vi "Single Slow IV v1.4.vi"() -> ()   [LabVIEW 2020]
uses:
  <vilib>/Utility/file.llb/Write Delimited Spreadsheet (DBL).vi
panel:
  out "Current variable":dbl
  in  "stop":bool
  in  "Tab Control 2":enum32{"cRIO plot", "Lockin X", "Lockin Y"}(tab)
  out "cRIO data plot":cluster{"Y":dbl[], "Y":dbl[]}[](graph)=[{"Y"=[0.1, 0.101, 0.10200000000000001, 0.10300000000000001, 0.10400000000000001, 0.10500000000000001, 0.10600000000000001, 0.10700000000000001, 0.10800000000000001, 0.10900000000000001, 0.11, 0.111, 0.112, 0.113, 0.114, 0.115, 0.116, 0.117, 0.11800000000000001, 0.11900000000000001, 0.12000000000000001, 0.12100000000000001, 0.122, 0.123, 0.124, 0.125, 0.126, 0.127, 0.128, 0.129, 0.13, 0.131, 0.132, 0.133, 0.134, 0.135, 0.136, 0.137, 0.138, 0.139, 0.14, 0.14100000000000001, 0.14200000000000002, 0.14300000000000002, 0.14400000000000002, 0.14500000000000002, 0.14600000000000002, 0.14700000000000002, 0.14800000000000002, 0.14900000000000002, 0.15000000000000002, 0.15100000000000002, 0.15200000000000002, 0.153, 0.154, 0.155, 0.156, 0.157, 0.158, 0.159, 0.16, 0.161, 0.162, 0.163, 0.164, 0.165, 0.166, 0.167, 0.168, 0.169, 0.17, 0.171, 0.17200000000000001, 0.173, 0.174, 0.175, 0.176, 0.177, 0.178, 0.179, 0.18, 0.181, 0.182, 0.183, 0.184, 0.185, 0.186, 0.187, 0.188, 0.189, 0.19, 0.191, 0.192, 0.193, 0.194, 0.195, 0.196, 0.197, 0.198, 0.199, 0.2], "Y"=[1.91443115234375e-05, 1.8234204101562503e-05, 1.8079296875e-05, 1.72965576171875e-05, 1.73908447265625e-05, 1.6982641601562502e-05, 1.7475024414062502e-05, 1.7350537109375e-05, 1.80681884765625e-05, 1.8036865234375e-05, 1.8520703124999998e-05, 1.9111669921875e-05, 1.948046875e-05, 1.9645117187500002e-05, 1.95529296875e-05, 1.9983398437500002e-05, 1.99129638671875e-05, 1.99599365234375e-05, 1.8666650390625e-05, 1.8764892578125e-05, 1.78889892578125e-05, 1.7660498046875002e-05, 1.7441210937500002e-05, 1.69652587890625e-05, 1.67341064453125e-05, 1.5950341796875e-05, 1.6491918945312503e-05, 1.61111572265625e-05, 1.6419482421875e-05, 1.6167163085937502e-05, 1.6684667968750002e-05, 1.66596923828125e-05, 1.76610595703125e-05, 1.7373608398437503e-05, 1.7419580078125e-05, 1.7511450195312502e-05, 1.76984619140625e-05, 1.7275e-05, 1.8423168945312502e-05, 1.78859619140625e-05, 1.74806396484375e-05, 1.7222802734375003e-05, 1.6946435546875e-05, 1.5935034179687498e-05, 1.5810864257812502e-05, 1.527841796875e-05, 1.509169921875e-05, 1.4530908203125001e-05, 1.4473876953125001e-05, 1.4885107421875e-05, 1.4928662109374999e-05, 1.5158349609375e-05, 1.5753149414062502e-05, 1.6247314453125003e-05, 1.59515625e-05, 1.62923583984375e-05, 1.64744873046875e-05, 1.65873779296875e-05, 1.7040673828125e-05, 1.65896484375e-05, 1.76021484375e-05, 1.6583422851562498e-05, 1.6492236328125e-05, 1.5975390625e-05, 1.57067138671875e-05, 1.4773681640625001e-05, 1.5178466796875001e-05, 1.4151171875e-05, 1.4718139648437501e-05, 1.453740234375e-05, 1.45205322265625e-05, 1.39417724609375e-05, 1.42656982421875e-05, 1.4501342773437501e-05, 1.4439892578125e-05, 1.47739501953125e-05, 1.47328369140625e-05, 1.46720703125e-05, 1.51514404296875e-05, 1.5362841796875e-05, 1.5647558593750002e-05, 1.612255859375e-05, 1.57461181640625e-05, 1.56584716796875e-05, 1.5264282226562502e-05, 1.4975024414062499e-05, 1.4608837890625003e-05, 1.4593286132812501e-05, 1.44783935546875e-05, 1.40139404296875e-05, 1.36931640625e-05, 1.3610986328125e-05, 1.3888769531250001e-05, 1.35940673828125e-05, 1.35070068359375e-05, 1.3863745117187502e-05, 1.45044677734375e-05, 1.418330078125e-05, 1.45068115234375e-05, 1.4514819335937501e-05, 1.4418505859375001e-05]}, {"Y"=[0.1, 0.101, 0.10200000000000001, 0.10300000000000001, 0.10400000000000001, 0.10500000000000001, 0.10600000000000001, 0.10700000000000001, 0.10800000000000001, 0.10900000000000001, 0.11, 0.111, 0.112, 0.113, 0.114, 0.115, 0.116, 0.117, 0.11800000000000001, 0.11900000000000001, 0.12000000000000001, 0.12100000000000001, 0.122, 0.123, 0.124, 0.125, 0.126, 0.127, 0.128, 0.129, 0.13, 0.131, 0.132, 0.133, 0.134, 0.135, 0.136, 0.137, 0.138, 0.139, 0.14, 0.14100000000000001, 0.14200000000000002, 0.14300000000000002, 0.14400000000000002, 0.14500000000000002, 0.14600000000000002, 0.14700000000000002, 0.14800000000000002, 0.14900000000000002, 0.15000000000000002, 0.15100000000000002, 0.15200000000000002, 0.153, 0.154, 0.155, 0.156, 0.157, 0.158, 0.159, 0.16, 0.161, 0.162, 0.163, 0.164, 0.165, 0.166, 0.167, 0.168, 0.169, 0.17, 0.171, 0.17200000000000001, 0.173, 0.174, 0.175, 0.176, 0.177, 0.178, 0.179, 0.18, 0.181, 0.182, 0.183, 0.184, 0.185, 0.186, 0.187, 0.188, 0.189, 0.19, 0.191, 0.192, 0.193, 0.194, 0.195, 0.196, 0.197, 0.198, 0.199, 0.2], "Y"=[2.07511962890625, 2.0750732421875, 2.074141357421875, 2.075462646484375, 2.075708740234375, 2.074308349609375, 2.074795654296875, 2.07555810546875, 2.0755185546875, 2.07468310546875, 2.074645751953125, 2.074962646484375, 2.0738427734375, 2.074322509765625, 2.07427294921875, 2.074574951171875, 2.075367431640625, 2.07494384765625, 2.074665771484375, 2.074663330078125, 2.07564013671875, 2.074562255859375, 2.074658935546875, 2.074733154296875, 2.07546826171875, 2.074733154296875, 2.074750244140625, 2.07523779296875, 2.07525244140625, 2.074369384765625, 2.075072265625, 2.0747587890625, 2.075584228515625, 2.075943603515625, 2.074529541015625, 2.07461474609375, 2.075067138671875, 2.075061279296875, 2.07536279296875, 2.07553466796875, 2.074748779296875, 2.075227294921875, 2.074936279296875, 2.075556396484375, 2.0753974609375, 2.0758994140625, 2.0761806640625, 2.075328369140625, 2.07436767578125, 2.076673828125, 2.076259765625, 2.075400146484375, 2.075468505859375, 2.075495849609375, 2.076040283203125, 2.0754658203125, 2.075578125, 2.0752451171875, 2.07488134765625, 2.07554736328125, 2.0753955078125, 2.0752822265625, 2.075176513671875, 2.076365478515625, 2.076373046875, 2.076056884765625, 2.07583837890625, 2.075223388671875, 2.0750703125, 2.07514599609375, 2.075769775390625, 2.0751220703125, 2.07619775390625, 2.075202392578125, 2.075671630859375, 2.07513916015625, 2.076079345703125, 2.076094970703125, 2.075864501953125, 2.07488134765625, 2.07613525390625, 2.076350341796875, 2.07625, 2.07523876953125, 2.075680419921875, 2.0746162109375, 2.076003173828125, 2.0753193359375, 2.075281494140625, 2.0755927734375, 2.075462158203125, 2.07468505859375, 2.07553564453125, 2.075280517578125, 2.0758173828125, 2.075341796875, 2.07434033203125, 2.074906005859375, 2.074229248046875, 2.0753671875, 2.0744853515625]}, {"Y"=[0.1, 0.101, 0.10200000000000001, 0.10300000000000001, 0.10400000000000001, 0.10500000000000001, 0.10600000000000001, 0.10700000000000001, 0.10800000000000001, 0.10900000000000001, 0.11, 0.111, 0.112, 0.113, 0.114, 0.115, 0.116, 0.117, 0.11800000000000001, 0.11900000000000001, 0.12000000000000001, 0.12100000000000001, 0.122, 0.123, 0.124, 0.125, 0.126, 0.127, 0.128, 0.129, 0.13, 0.131, 0.132, 0.133, 0.134, 0.135, 0.136, 0.137, 0.138, 0.139, 0.14, 0.14100000000000001, 0.14200000000000002, 0.14300000000000002, 0.14400000000000002, 0.14500000000000002, 0.14600000000000002, 0.14700000000000002, 0.14800000000000002, 0.14900000000000002, 0.15000000000000002, 0.15100000000000002, 0.15200000000000002, 0.153, 0.154, 0.155, 0.156, 0.157, 0.158, 0.159, 0.16, 0.161, 0.162, 0.163, 0.164, 0.165, 0.166, 0.167, 0.168, 0.169, 0.17, 0.171, 0.17200000000000001, 0.173, 0.174, 0.175, 0.176, 0.177, 0.178, 0.179, 0.18, 0.181, 0.182, 0.183, 0.184, 0.185, 0.186, 0.187, 0.188, 0.189, 0.19, 0.191, 0.192, 0.193, 0.194, 0.195, 0.196, 0.197, 0.198, 0.199, 0.2], "Y"=[0.000849365234375, 0.0008095703125, 0.000814453125, 0.00078076171875, 0.000771240234375, 0.000831787109375, 0.000755859375, 0.00079150390625, 0.0008310546875, 0.00079150390625, 0.00074560546875, 0.00078369140625, 0.000753662109375, 0.00079296875, 0.0007275390625, 0.000805419921875, 0.00074658203125, 0.00084375, 0.000741943359375, 0.00080859375, 0.00072705078125, 0.0007802734375, 0.0007021484375, 0.0008046875, 0.000873779296875, 0.000772216796875, 0.0007861328125, 0.000777587890625, 0.00078466796875, 0.00077001953125, 0.000764404296875, 0.0007626953125, 0.000732421875, 0.00077783203125, 0.00079150390625, 0.0007861328125, 0.000770751953125, 0.0008134765625, 0.00080419921875, 0.00079345703125, 0.000803466796875, 0.0007470703125, 0.000757080078125, 0.000783935546875, 0.000799072265625, 0.000781982421875, 0.00076904296875, 0.000742919921875, 0.00082666015625, 0.00078369140625, 0.000858154296875, 0.00076318359375, 0.0006982421875, 0.00071728515625, 0.00077099609375, 0.00078076171875, 0.000766845703125, 0.00076806640625, 0.000752197265625, 0.000720703125, 0.00075830078125, 0.00077099609375, 0.0008076171875, 0.000795166015625, 0.00074365234375, 0.000795166015625, 0.00078125, 0.000791748046875, 0.000809814453125, 0.00074755859375, 0.000774658203125, 0.000756103515625, 0.00083251953125, 0.000758056640625, 0.00082470703125, 0.00077197265625, 0.000834228515625, 0.000770751953125, 0.00077734375, 0.000760009765625, 0.000823974609375, 0.00071533203125, 0.000766357421875, 0.0007548828125, 0.000796630859375, 0.000743408203125, 0.000770751953125, 0.000744384765625, 0.0007314453125, 0.000734130859375, 0.000804443359375, 0.0007275390625, 0.000815673828125, 0.000766357421875, 0.000784912109375, 0.000762451171875, 0.00075, 0.000779296875, 0.000757080078125, 0.000751953125, 0.000764892578125]}, {"Y"=[0.1, 0.101, 0.10200000000000001, 0.10300000000000001, 0.10400000000000001, 0.10500000000000001, 0.10600000000000001, 0.10700000000000001, 0.10800000000000001, 0.10900000000000001, 0.11, 0.111, 0.112, 0.113, 0.114, 0.115, 0.116, 0.117, 0.11800000000000001, 0.11900000000000001, 0.12000000000000001, 0.12100000000000001, 0.122, 0.123, 0.124, 0.125, 0.126, 0.127, 0.128, 0.129, 0.13, 0.131, 0.132, 0.133, 0.134, 0.135, 0.136, 0.137, 0.138, 0.139, 0.14, 0.14100000000000001, 0.14200000000000002, 0.14300000000000002, 0.14400000000000002, 0.14500000000000002, 0.14600000000000002, 0.14700000000000002, 0.14800000000000002, 0.14900000000000002, 0.15000000000000002, 0.15100000000000002, 0.15200000000000002, 0.153, 0.154, 0.155, 0.156, 0.157, 0.158, 0.159, 0.16, 0.161, 0.162, 0.163, 0.164, 0.165, 0.166, 0.167, 0.168, 0.169, 0.17, 0.171, 0.17200000000000001, 0.173, 0.174, 0.175, 0.176, 0.177, 0.178, 0.179, 0.18, 0.181, 0.182, 0.183, 0.184, 0.185, 0.186, 0.187, 0.188, 0.189, 0.19, 0.191, 0.192, 0.193, 0.194, 0.195, 0.196, 0.197, 0.198, 0.199, 0.2], "Y"=[0.00172021484375, 0.001699462890625, 0.001721435546875, 0.001740966796875, 0.001722412109375, 0.001780517578125, 0.001792724609375, 0.00180224609375, 0.001711181640625, 0.00181494140625, 0.001773193359375, 0.001771240234375, 0.00173388671875, 0.001708740234375, 0.00180908203125, 0.001841064453125, 0.001756103515625, 0.00170068359375, 0.00175, 0.001714111328125, 0.001801025390625, 0.001765625, 0.0017099609375, 0.001703857421875, 0.001786865234375, 0.0018046875, 0.001700927734375, 0.001765380859375, 0.001693603515625, 0.00175244140625, 0.0017626953125, 0.0017978515625, 0.001715576171875, 0.001716064453125, 0.00177099609375, 0.00180712890625, 0.001722900390625, 0.001816650390625, 0.001749755859375, 0.00174755859375, 0.001776123046875, 0.00170849609375, 0.00172509765625, 0.001736083984375, 0.00171533203125, 0.001705322265625, 0.001744873046875, 0.001779296875, 0.001696044921875, 0.00173974609375, 0.001815185546875, 0.001720947265625, 0.00178076171875, 0.001763916015625, 0.0017958984375, 0.0017158203125, 0.00179248046875, 0.001754638671875, 0.00173193359375, 0.001706298828125, 0.00173388671875, 0.00166943359375, 0.0017373046875, 0.001741943359375, 0.001747314453125, 0.001755615234375, 0.001791748046875, 0.001772216796875, 0.001737548828125, 0.00176904296875, 0.00175830078125, 0.001655029296875, 0.001769775390625, 0.001682861328125, 0.00176318359375, 0.00177294921875, 0.00177001953125, 0.00178271484375, 0.00175537109375, 0.00174755859375, 0.001724365234375, 0.001774658203125, 0.0017412109375, 0.001767333984375, 0.00175341796875, 0.0017685546875, 0.0017138671875, 0.0017158203125, 0.00172998046875, 0.001653076171875, 0.0017529296875, 0.001751708984375, 0.001750244140625, 0.00172265625, 0.00180859375, 0.00176953125, 0.00177490234375, 0.001733154296875, 0.001750244140625, 0.001706298828125, 0.0017529296875]}]
  out "cRIO Plot 0":string="DC Voltage V"
  out "cRIO Plot 1":string="DC current uA"
  out "cRIO Plot 2":string="dV V"
  out "cRIO Plot 3":string="dI uA"
  out "Lockin X":cluster{"Y":dbl[], "Y":dbl[]}[](graph)=[{"Y"=[0.1, 0.101, 0.10200000000000001, 0.10300000000000001, 0.10400000000000001, 0.10500000000000001, 0.10600000000000001, 0.10700000000000001, 0.10800000000000001, 0.10900000000000001, 0.11, 0.111, 0.112, 0.113, 0.114, 0.115, 0.116, 0.117, 0.11800000000000001, 0.11900000000000001, 0.12000000000000001, 0.12100000000000001, 0.122, 0.123, 0.124, 0.125, 0.126, 0.127, 0.128, 0.129, 0.13, 0.131, 0.132, 0.133, 0.134, 0.135, 0.136, 0.137, 0.138, 0.139, 0.14, 0.14100000000000001, 0.14200000000000002, 0.14300000000000002, 0.14400000000000002, 0.14500000000000002, 0.14600000000000002, 0.14700000000000002, 0.14800000000000002, 0.14900000000000002, 0.15000000000000002, 0.15100000000000002, 0.15200000000000002, 0.153, 0.154, 0.155, 0.156, 0.157, 0.158, 0.159, 0.16, 0.161, 0.162, 0.163, 0.164, 0.165, 0.166, 0.167, 0.168, 0.169, 0.17, 0.171, 0.17200000000000001, 0.173, 0.174, 0.175, 0.176, 0.177, 0.178, 0.179, 0.18, 0.181, 0.182, 0.183, 0.184, 0.185, 0.186, 0.187, 0.188, 0.189, 0.19, 0.191, 0.192, 0.193, 0.194, 0.195, 0.196, 0.197, 0.198, 0.199, 0.2], "Y"=[1.41335, 1.26267, 0.92316, 1.13488, 1.13869, 1.297, 1.30273, 1.3466, 1.35041, 1.09673, 1.13679, 1.0013699999999999, 1.02998, 1.0681200000000002, 0.974659, 0.8926430000000001, 1.33706, 1.05477, 1.02235, 1.29319, 1.03951, 1.3141699999999998, 1.31989, 1.35613, 1.07766, 0.74387, 0.795368, 0.93079, 0.812534, 0.8869210000000001, 1.02235, 1.12153, 1.23788, 1.0585900000000001, 1.02807, 0.928883, 1.13488, 0.9727520000000001, 0.86594, 0.856403, 0.812534, 0.8754770000000001, 1.0604900000000002, 0.963215, 0.957493, 1.00899, 1.08147, 0.8697550000000001, 0.974659, 1.14632, 1.0585900000000001, 0.963215, 0.633243, 0.770573, 1.03761, 0.911716, 0.9594, 1.08529, 1.10436, 1.07766, 0.822071, 0.879291, 1.11008, 1.17493, 1.05477, 0.909809, 0.720982, 0.629429, 0.698093, 0.909809, 0.967029, 0.913624, 0.92316, 0.810627, 0.949863, 1.07384, 1.14823, 1.22262, 1.0662200000000002, 1.01281, 0.8697550000000001, 1.0604900000000002, 0.9594, 0.734333, 0.8316079999999999, 0.835422, 0.8964580000000001, 0.764851, 0.804905, 0.791553, 0.947956, 0.5817450000000001, 0.654224, 0.625614, 0.631336, 0.711445, 0.730518, 0.606541, 0.633243, 0.703815, 0.646595]}, {"Y"=[0.1, 0.101, 0.10200000000000001, 0.10300000000000001, 0.10400000000000001, 0.10500000000000001, 0.10600000000000001, 0.10700000000000001, 0.10800000000000001, 0.10900000000000001, 0.11, 0.111, 0.112, 0.113, 0.114, 0.115, 0.116, 0.117, 0.11800000000000001, 0.11900000000000001, 0.12000000000000001, 0.12100000000000001, 0.122, 0.123, 0.124, 0.125, 0.126, 0.127, 0.128, 0.129, 0.13, 0.131, 0.132, 0.133, 0.134, 0.135, 0.136, 0.137, 0.138, 0.139, 0.14, 0.14100000000000001, 0.14200000000000002, 0.14300000000000002, 0.14400000000000002, 0.14500000000000002, 0.14600000000000002, 0.14700000000000002, 0.14800000000000002, 0.14900000000000002, 0.15000000000000002, 0.15100000000000002, 0.15200000000000002, 0.153, 0.154, 0.155, 0.156, 0.157, 0.158, 0.159, 0.16, 0.161, 0.162, 0.163, 0.164, 0.165, 0.166, 0.167, 0.168, 0.169, 0.17, 0.171, 0.17200000000000001, 0.173, 0.174, 0.175, 0.176, 0.177, 0.178, 0.179, 0.18, 0.181, 0.182, 0.183, 0.184, 0.185, 0.186, 0.187, 0.188, 0.189, 0.19, 0.191, 0.192, 0.193, 0.194, 0.195, 0.196, 0.197, 0.198, 0.199, 0.2], "Y"=[0.755314, 0.915531, 0.9594, 0.967029, 0.9727520000000001, 0.970844, 0.970844, 0.974659, 0.970844, 0.974659, 0.974659, 0.974659, 0.9727520000000001, 0.9727520000000001, 0.974659, 0.970844, 0.9727520000000001, 0.9765699999999999, 0.9765699999999999, 0.9765699999999999, 0.974659, 0.9765699999999999, 0.9803850000000001, 0.9765699999999999, 0.9765699999999999, 0.974659, 0.9727520000000001, 0.9727520000000001, 0.9727520000000001, 0.9765699999999999, 0.974659, 0.9784769999999999, 0.9784769999999999, 0.974659, 0.968937, 0.967029, 0.970844, 0.9765699999999999, 0.9765699999999999, 0.974659, 0.9727520000000001, 0.9727520000000001, 0.9765699999999999, 0.9765699999999999, 0.9765699999999999, 0.974659, 0.9765699999999999, 0.9765699999999999, 0.9765699999999999, 0.9727520000000001, 0.9727520000000001, 0.9765699999999999, 0.9803850000000001, 0.982292, 0.9784769999999999, 0.9784769999999999, 0.974659, 0.974659, 0.9765699999999999, 0.974659, 0.974659, 0.9727520000000001, 0.9765699999999999, 0.9784769999999999, 0.984199, 0.982292, 0.9765699999999999, 0.9765699999999999, 0.974659, 0.974659, 0.9765699999999999, 0.9765699999999999, 0.9765699999999999, 0.9784769999999999, 0.9765699999999999, 0.9765699999999999, 0.9765699999999999, 0.9765699999999999, 0.974659, 0.9765699999999999, 0.9765699999999999, 0.9765699999999999, 0.970844, 0.970844, 0.9765699999999999, 0.9727520000000001, 0.970844, 0.968937, 0.9727520000000001, 0.9765699999999999, 0.9765699999999999, 0.9784769999999999, 0.9765699999999999, 0.9765699999999999, 0.9765699999999999, 0.9765699999999999, 0.9727520000000001, 0.968937, 0.968937, 0.967029, 0.9727520000000001]}, {"Y"=[0.1, 0.101, 0.10200000000000001, 0.10300000000000001, 0.10400000000000001, 0.10500000000000001, 0.10600000000000001, 0.10700000000000001, 0.10800000000000001, 0.10900000000000001, 0.11, 0.111, 0.112, 0.113, 0.114, 0.115, 0.116, 0.117, 0.11800000000000001, 0.11900000000000001, 0.12000000000000001, 0.12100000000000001, 0.122, 0.123, 0.124, 0.125, 0.126, 0.127, 0.128, 0.129, 0.13, 0.131, 0.132, 0.133, 0.134, 0.135, 0.136, 0.137, 0.138, 0.139, 0.14, 0.14100000000000001, 0.14200000000000002, 0.14300000000000002, 0.14400000000000002, 0.14500000000000002, 0.14600000000000002, 0.14700000000000002, 0.14800000000000002, 0.14900000000000002, 0.15000000000000002, 0.15100000000000002, 0.15200000000000002, 0.153, 0.154, 0.155, 0.156, 0.157, 0.158, 0.159, 0.16, 0.161, 0.162, 0.163, 0.164, 0.165, 0.166, 0.167, 0.168, 0.169, 0.17, 0.171, 0.17200000000000001, 0.173, 0.174, 0.175, 0.176, 0.177, 0.178, 0.179, 0.18, 0.181, 0.182, 0.183, 0.184, 0.185, 0.186, 0.187, 0.188, 0.189, 0.19, 0.191, 0.192, 0.193, 0.194, 0.195, 0.196, 0.197, 0.198, 0.199, 0.2], "Y"=[0.0, 0.0, 0.0, 0.0, 0.0, 0.0, 0.0, 0.0, 0.0, 0.0, 0.0, 0.0, 0.0, 0.0, 0.0, 0.0, 0.0, 0.0, 0.0, 0.0, 0.0, 0.0, 0.0, 0.0, 0.0, 0.0, 0.0, 0.0, 0.0, 0.0, 0.0, 0.0, 0.0, 0.0, 0.0, 0.0, 0.0, 0.0, 0.0, 0.0, 0.0, 0.0, 0.0, 0.0, 0.0, 0.0, 0.0, 0.0, 0.0, 0.0, 0.0, 0.0, 0.0, 0.0, 0.0, 0.0, 0.0, 0.0, 0.0, 0.0, 0.0, 0.0, 0.0, 0.0, 0.0, 0.0, 0.0, 0.0, 0.0, 0.0, 0.0, 0.0, 0.0, 0.0, 0.0, 0.0, 0.0, 0.0, 0.0, 0.0, 0.0, 0.0, 0.0, 0.0, 0.0, 0.0, 0.0, 0.0, 0.0, 0.0, 0.0, 0.0, 0.0, 0.0, 0.0, 0.0, 0.0, 0.0, 0.0, 0.0, 0.0]}, {"Y"=[0.1, 0.101, 0.10200000000000001, 0.10300000000000001, 0.10400000000000001, 0.10500000000000001, 0.10600000000000001, 0.10700000000000001, 0.10800000000000001, 0.10900000000000001, 0.11, 0.111, 0.112, 0.113, 0.114, 0.115, 0.116, 0.117, 0.11800000000000001, 0.11900000000000001, 0.12000000000000001, 0.12100000000000001, 0.122, 0.123, 0.124, 0.125, 0.126, 0.127, 0.128, 0.129, 0.13, 0.131, 0.132, 0.133, 0.134, 0.135, 0.136, 0.137, 0.138, 0.139, 0.14, 0.14100000000000001, 0.14200000000000002, 0.14300000000000002, 0.14400000000000002, 0.14500000000000002, 0.14600000000000002, 0.14700000000000002, 0.14800000000000002, 0.14900000000000002, 0.15000000000000002, 0.15100000000000002, 0.15200000000000002, 0.153, 0.154, 0.155, 0.156, 0.157, 0.158, 0.159, 0.16, 0.161, 0.162, 0.163, 0.164, 0.165, 0.166, 0.167, 0.168, 0.169, 0.17, 0.171, 0.17200000000000001, 0.173, 0.174, 0.175, 0.176, 0.177, 0.178, 0.179, 0.18, 0.181, 0.182, 0.183, 0.184, 0.185, 0.186, 0.187, 0.188, 0.189, 0.19, 0.191, 0.192, 0.193, 0.194, 0.195, 0.196, 0.197, 0.198, 0.199, 0.2], "Y"=[0.0, 0.0, 0.0, 0.0, 0.0, 0.0, 0.0, 0.0, 0.0, 0.0, 0.0, 0.0, 0.0, 0.0, 0.0, 0.0, 0.0, 0.0, 0.0, 0.0, 0.0, 0.0, 0.0, 0.0, 0.0, 0.0, 0.0, 0.0, 0.0, 0.0, 0.0, 0.0, 0.0, 0.0, 0.0, 0.0, 0.0, 0.0, 0.0, 0.0, 0.0, 0.0, 0.0, 0.0, 0.0, 0.0, 0.0, 0.0, 0.0, 0.0, 0.0, 0.0, 0.0, 0.0, 0.0, 0.0, 0.0, 0.0, 0.0, 0.0, 0.0, 0.0, 0.0, 0.0, 0.0, 0.0, 0.0, 0.0, 0.0, 0.0, 0.0, 0.0, 0.0, 0.0, 0.0, 0.0, 0.0, 0.0, 0.0, 0.0, 0.0, 0.0, 0.0, 0.0, 0.0, 0.0, 0.0, 0.0, 0.0, 0.0, 0.0, 0.0, 0.0, 0.0, 0.0, 0.0, 0.0, 0.0, 0.0, 0.0, 0.0]}]
  out "Lockin Y":cluster{"Y":dbl[], "Y":dbl[]}[](graph)=[{"Y"=[0.1, 0.101, 0.10200000000000001, 0.10300000000000001, 0.10400000000000001, 0.10500000000000001, 0.10600000000000001, 0.10700000000000001, 0.10800000000000001, 0.10900000000000001, 0.11, 0.111, 0.112, 0.113, 0.114, 0.115, 0.116, 0.117, 0.11800000000000001, 0.11900000000000001, 0.12000000000000001, 0.12100000000000001, 0.122, 0.123, 0.124, 0.125, 0.126, 0.127, 0.128, 0.129, 0.13, 0.131, 0.132, 0.133, 0.134, 0.135, 0.136, 0.137, 0.138, 0.139, 0.14, 0.14100000000000001, 0.14200000000000002, 0.14300000000000002, 0.14400000000000002, 0.14500000000000002, 0.14600000000000002, 0.14700000000000002, 0.14800000000000002, 0.14900000000000002, 0.15000000000000002, 0.15100000000000002, 0.15200000000000002, 0.153, 0.154, 0.155, 0.156, 0.157, 0.158, 0.159, 0.16, 0.161, 0.162, 0.163, 0.164, 0.165, 0.166, 0.167, 0.168, 0.169, 0.17, 0.171, 0.17200000000000001, 0.173, 0.174, 0.175, 0.176, 0.177, 0.178, 0.179, 0.18, 0.181, 0.182, 0.183, 0.184, 0.185, 0.186, 0.187, 0.188, 0.189, 0.19, 0.191, 0.192, 0.193, 0.194, 0.195, 0.196, 0.197, 0.198, 0.199, 0.2], "Y"=[-0.349047, -0.234605, -0.135423, -0.265123, -0.20408700000000002, -0.144959, -0.106812, 0.0953679, -0.0953679, -0.5397829999999999, -0.608448, -0.364305, -0.33951000000000003, -0.38337899999999997, -0.261309, -0.08010909999999999, 0.0114442, -0.0877385, 0.164033, 0.0381472, -0.034332499999999995, -0.265123, -0.0915532, -0.026703, -0.0953679, -0.06866499999999999, -0.17357, -0.27275299999999997, -0.270845, -0.17357, -0.0762944, -0.23842000000000002, -0.253679, -0.175477, -0.316622, 0.0839238, -0.0743871, -0.278475, -0.164033, -0.23079, -0.305178, -0.33188100000000004, -0.234605, -0.16975500000000002, -0.278475, -0.146867, -0.186921, -0.389101, -0.411989, -0.349047, -0.20790199999999998, -0.026703, -0.26893799999999995, -0.13732999999999998, 0.0743871, -0.020981, -0.0667577, -0.156404, -0.167848, 0.110627, 0.400545, 0.16975500000000002, -0.118256, -0.034332499999999995, 0.108719, 0.167848, 0.127793, 0.07247970000000001, 0.062943, 0.0915532, 0.0839238, -0.0171663, 0.0572207, 0.053406, -0.23079, -0.16594, -0.307085, -0.379564, -0.118256, -0.125886, -0.183106, -0.125886, 0.0419619, -0.0667577, -0.055313299999999996, -0.059128, 0.034332499999999995, 0.0610356, -0.116349, -0.144959, -0.24605, -0.240327, -0.318529, -0.352861, -0.356676, -0.110627, -0.102997, -0.0972752, 0.20408700000000002, 0.144959, 0.20218]}, {"Y"=[0.1, 0.101, 0.10200000000000001, 0.10300000000000001, 0.10400000000000001, 0.10500000000000001, 0.10600000000000001, 0.10700000000000001, 0.10800000000000001, 0.10900000000000001, 0.11, 0.111, 0.112, 0.113, 0.114, 0.115, 0.116, 0.117, 0.11800000000000001, 0.11900000000000001, 0.12000000000000001, 0.12100000000000001, 0.122, 0.123, 0.124, 0.125, 0.126, 0.127, 0.128, 0.129, 0.13, 0.131, 0.132, 0.133, 0.134, 0.135, 0.136, 0.137, 0.138, 0.139, 0.14, 0.14100000000000001, 0.14200000000000002, 0.14300000000000002, 0.14400000000000002, 0.14500000000000002, 0.14600000000000002, 0.14700000000000002, 0.14800000000000002, 0.14900000000000002, 0.15000000000000002, 0.15100000000000002, 0.15200000000000002, 0.153, 0.154, 0.155, 0.156, 0.157, 0.158, 0.159, 0.16, 0.161, 0.162, 0.163, 0.164, 0.165, 0.166, 0.167, 0.168, 0.169, 0.17, 0.171, 0.17200000000000001, 0.173, 0.174, 0.175, 0.176, 0.177, 0.178, 0.179, 0.18, 0.181, 0.182, 0.183, 0.184, 0.185, 0.186, 0.187, 0.188, 0.189, 0.19, 0.191, 0.192, 0.193, 0.194, 0.195, 0.196, 0.197, 0.198, 0.199, 0.2], "Y"=[-0.20790199999999998, -0.114441, -0.0915532, -0.0858312, -0.08010909999999999, -0.0820165, -0.0858312, -0.0839238, -0.0858312, -0.0858312, -0.0858312, -0.0896459, -0.0839238, -0.0858312, -0.0858312, -0.0877385, -0.0877385, -0.0839238, -0.0820165, -0.0858312, -0.0820165, -0.0839238, -0.0858312, -0.0896459, -0.0915532, -0.0877385, -0.0839238, -0.0877385, -0.0877385, -0.0820165, -0.0839238, -0.0820165, -0.0839238, -0.0839238, -0.08010909999999999, -0.0839238, -0.0820165, -0.0877385, -0.0839238, -0.0858312, -0.0858312, -0.0820165, -0.0820165, -0.08010909999999999, -0.0877385, -0.0915532, -0.0934605, -0.0877385, -0.0820165, -0.08010909999999999, -0.08010909999999999, -0.0858312, -0.0820165, -0.0820165, -0.0896459, -0.0877385, -0.0877385, -0.0858312, -0.0839238, -0.08010909999999999, -0.0858312, -0.0839238, -0.08010909999999999, -0.08010909999999999, -0.0839238, -0.08010909999999999, -0.0839238, -0.0877385, -0.0915532, -0.0858312, -0.0839238, -0.0858312, -0.0896459, -0.0915532, -0.0877385, -0.0839238, -0.08010909999999999, -0.08010909999999999, -0.0820165, -0.0820165, -0.0839238, -0.08010909999999999, -0.0839238, -0.0858312, -0.0858312, -0.0915532, -0.0896459, -0.0820165, -0.07820179999999999, -0.08010909999999999, -0.0820165, -0.08010909999999999, -0.0762944, -0.0820165, -0.0820165, -0.0858312, -0.0820165, -0.08010909999999999, -0.0858312, -0.0896459, -0.0877385]}, {"Y"=[0.1, 0.101, 0.10200000000000001, 0.10300000000000001, 0.10400000000000001, 0.10500000000000001, 0.10600000000000001, 0.10700000000000001, 0.10800000000000001, 0.10900000000000001, 0.11, 0.111, 0.112, 0.113, 0.114, 0.115, 0.116, 0.117, 0.11800000000000001, 0.11900000000000001, 0.12000000000000001, 0.12100000000000001, 0.122, 0.123, 0.124, 0.125, 0.126, 0.127, 0.128, 0.129, 0.13, 0.131, 0.132, 0.133, 0.134, 0.135, 0.136, 0.137, 0.138, 0.139, 0.14, 0.14100000000000001, 0.14200000000000002, 0.14300000000000002, 0.14400000000000002, 0.14500000000000002, 0.14600000000000002, 0.14700000000000002, 0.14800000000000002, 0.14900000000000002, 0.15000000000000002, 0.15100000000000002, 0.15200000000000002, 0.153, 0.154, 0.155, 0.156, 0.157, 0.158, 0.159, 0.16, 0.161, 0.162, 0.163, 0.164, 0.165, 0.166, 0.167, 0.168, 0.169, 0.17, 0.171, 0.17200000000000001, 0.173, 0.174, 0.175, 0.176, 0.177, 0.178, 0.179, 0.18, 0.181, 0.182, 0.183, 0.184, 0.185, 0.186, 0.187, 0.188, 0.189, 0.19, 0.191, 0.192, 0.193, 0.194, 0.195, 0.196, 0.197, 0.198, 0.199, 0.2], "Y"=[0.0, 0.0, 0.0, 0.0, 0.0, 0.0, 0.0, 0.0, 0.0, 0.0, 0.0, 0.0, 0.0, 0.0, 0.0, 0.0, 0.0, 0.0, 0.0, 0.0, 0.0, 0.0, 0.0, 0.0, 0.0, 0.0, 0.0, 0.0, 0.0, 0.0, 0.0, 0.0, 0.0, 0.0, 0.0, 0.0, 0.0, 0.0, 0.0, 0.0, 0.0, 0.0, 0.0, 0.0, 0.0, 0.0, 0.0, 0.0, 0.0, 0.0, 0.0, 0.0, 0.0, 0.0, 0.0, 0.0, 0.0, 0.0, 0.0, 0.0, 0.0, 0.0, 0.0, 0.0, 0.0, 0.0, 0.0, 0.0, 0.0, 0.0, 0.0, 0.0, 0.0, 0.0, 0.0, 0.0, 0.0, 0.0, 0.0, 0.0, 0.0, 0.0, 0.0, 0.0, 0.0, 0.0, 0.0, 0.0, 0.0, 0.0, 0.0, 0.0, 0.0, 0.0, 0.0, 0.0, 0.0, 0.0, 0.0, 0.0, 0.0]}, {"Y"=[0.1, 0.101, 0.10200000000000001, 0.10300000000000001, 0.10400000000000001, 0.10500000000000001, 0.10600000000000001, 0.10700000000000001, 0.10800000000000001, 0.10900000000000001, 0.11, 0.111, 0.112, 0.113, 0.114, 0.115, 0.116, 0.117, 0.11800000000000001, 0.11900000000000001, 0.12000000000000001, 0.12100000000000001, 0.122, 0.123, 0.124, 0.125, 0.126, 0.127, 0.128, 0.129, 0.13, 0.131, 0.132, 0.133, 0.134, 0.135, 0.136, 0.137, 0.138, 0.139, 0.14, 0.14100000000000001, 0.14200000000000002, 0.14300000000000002, 0.14400000000000002, 0.14500000000000002, 0.14600000000000002, 0.14700000000000002, 0.14800000000000002, 0.14900000000000002, 0.15000000000000002, 0.15100000000000002, 0.15200000000000002, 0.153, 0.154, 0.155, 0.156, 0.157, 0.158, 0.159, 0.16, 0.161, 0.162, 0.163, 0.164, 0.165, 0.166, 0.167, 0.168, 0.169, 0.17, 0.171, 0.17200000000000001, 0.173, 0.174, 0.175, 0.176, 0.177, 0.178, 0.179, 0.18, 0.181, 0.182, 0.183, 0.184, 0.185, 0.186, 0.187, 0.188, 0.189, 0.19, 0.191, 0.192, 0.193, 0.194, 0.195, 0.196, 0.197, 0.198, 0.199, 0.2], "Y"=[0.0, 0.0, 0.0, 0.0, 0.0, 0.0, 0.0, 0.0, 0.0, 0.0, 0.0, 0.0, 0.0, 0.0, 0.0, 0.0, 0.0, 0.0, 0.0, 0.0, 0.0, 0.0, 0.0, 0.0, 0.0, 0.0, 0.0, 0.0, 0.0, 0.0, 0.0, 0.0, 0.0, 0.0, 0.0, 0.0, 0.0, 0.0, 0.0, 0.0, 0.0, 0.0, 0.0, 0.0, 0.0, 0.0, 0.0, 0.0, 0.0, 0.0, 0.0, 0.0, 0.0, 0.0, 0.0, 0.0, 0.0, 0.0, 0.0, 0.0, 0.0, 0.0, 0.0, 0.0, 0.0, 0.0, 0.0, 0.0, 0.0, 0.0, 0.0, 0.0, 0.0, 0.0, 0.0, 0.0, 0.0, 0.0, 0.0, 0.0, 0.0, 0.0, 0.0, 0.0, 0.0, 0.0, 0.0, 0.0, 0.0, 0.0, 0.0, 0.0, 0.0, 0.0, 0.0, 0.0, 0.0, 0.0, 0.0, 0.0, 0.0]}]
  in  "Tab Control":enum32{"cRIO", "variable", "Lockin", "Status"}(tab)=enum."variable"
  in  "cRIO Chan 0":bool=TRUE
  in  "cRIO IP":string="//172.22.11.2"
  in  "Reading Average times":i32=1000
  in  "read cRIO":bool=TRUE
  in  "Scale factor3":dbl=1.0
  in  "Channel name 3":string(combo)="dI uA"
  in  "cRIO Chan 3":bool
  in  "Scale factor2":dbl=1.0
  in  "Channel name 2":string(combo)="dV V"
  in  "cRIO Chan 2":bool
  in  "Scale factor1":dbl=1.0
  in  "Channel name 1":string(combo)="DC current uA"
  in  "cRIO Chan 1":bool=TRUE
  in  "Scale factor0":dbl=0.0001
  in  "Channel name 0":string(combo)="DC Voltage V"
  out "Unit":string="mT"
  in  "Tab for variable":enum32{"Current", "Magnetic field"}(tab)=enum."Magnetic field"
  in  "Delay Time s":dbl=1.5 caption="Delay Time (s)"
  in  "AO Channel":string(combo)="AO0"
  in  "current output Scale factor":dbl=1.0
  in  "Fixed current uA":dbl=2.1
  in  "Scale factor":dbl=1.0
  in  "Field Rate mT per sec":dbl=0.1 format="%#_13g"
  in  "Magnet Device Select":string(combo)="NI DAQ Controlled V to I source"
  in  "Start":dbl=0.1
  in  "Range":dbl=0.1
  in  "Step":dbl=0.001
  in  "Ramp type":string(combo)="Range"
  in  "Ramp up first T":bool=TRUE
  in  "Lockin address 4":string
  in  "Lockin address 3":string
  in  "Lockin address 2":string="GPIB0::9::INSTR"
  in  "Lockin address 1":string="GPIB0::8::INSTR"
  in  "Lockin 4":bool
  in  "Lockin 3":bool
  in  "Lockin 2":bool=TRUE
  in  "Lockin 1":bool=TRUE
  in  "Use Lockin":bool=TRUE
  in  "Lockin Chan name 4":string(combo)="None"
  in  "Lockin Chan name 3":string(combo)="None"
  in  "Lockin Chan name 2":string(combo)="Current mV"
  in  "Lockin Chan name 1":string(combo)="Voltage mV"
  in  "Lockin and field and temperature status":string="Data File time stamp 20210723-212111\nTemperature Chan1 1.218210, Chan2 0.050013\nmagnetic field InfmT\nLockin status\n#Device channel name Voltage mV#Device \u0000\u0000\u0000\u000fGPIB0::8::INSTR\n #PHASE=0\n #REF=1\n #FREQ=17\n #INPUT=0\n #SENS=22\n #TIMECONST=10\n #VOLTAGE=0.1\n#Device channel name Current mV#Device \u0000\u0000\u0000\u000fGPIB0::9::INSTR\n #PHASE=0\n #REF=0\n #FREQ=16.9997\n #INPUT=0\n #SENS=22\n #TIMECONST=10\n #VOLTAGE=0.004\n"
  in  "Temp Device":string(combo)="Elsa"
  in  "Temp Chan1":string="T5"
  in  "Temp Chan2":string="T8"
  in  "Magnetic field read device":string(combo)="Elsa Magnet"
  in  "Record Field":bool
  in  "Contour plot folder":path=path "C:/Users/gyue/Desktop/Data folder 20210720"
  out "error out":errorcluster
  # "Voltage x factor=actual"
  # "Voltage x factor=uA"
  # "Voltage x factor=uA"
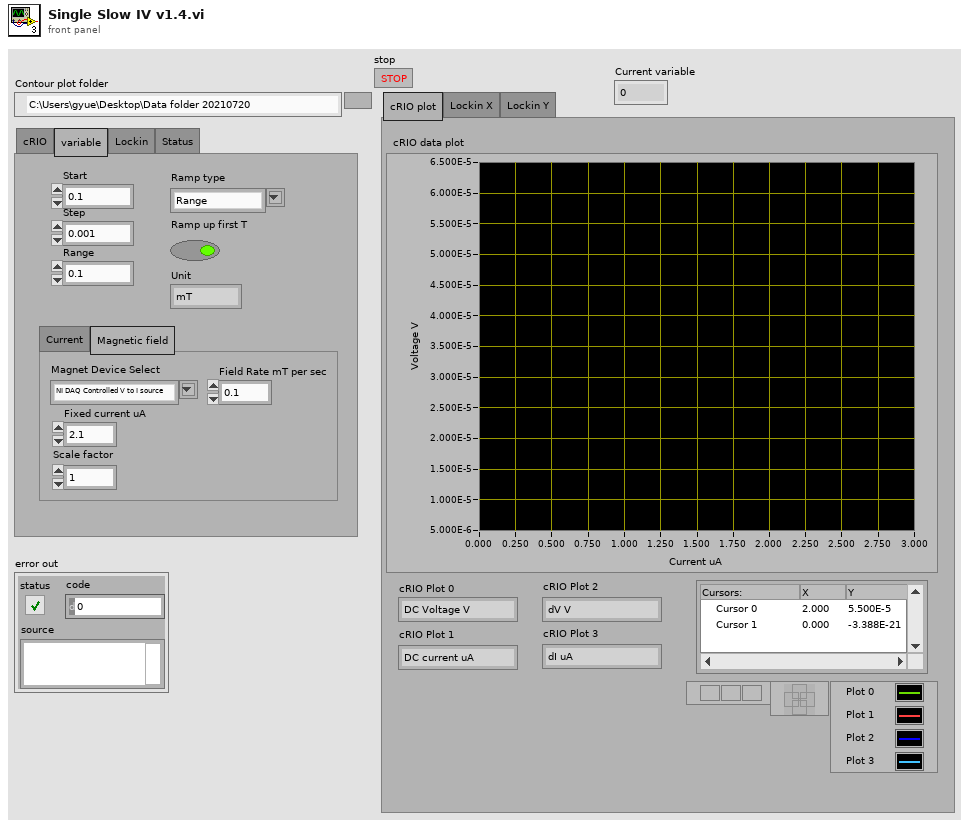
[diagram p1: front panel]
types:
  T1 = cluster{"AI0":dbl, "AI1":dbl, "AI2":dbl, "AI3":dbl}
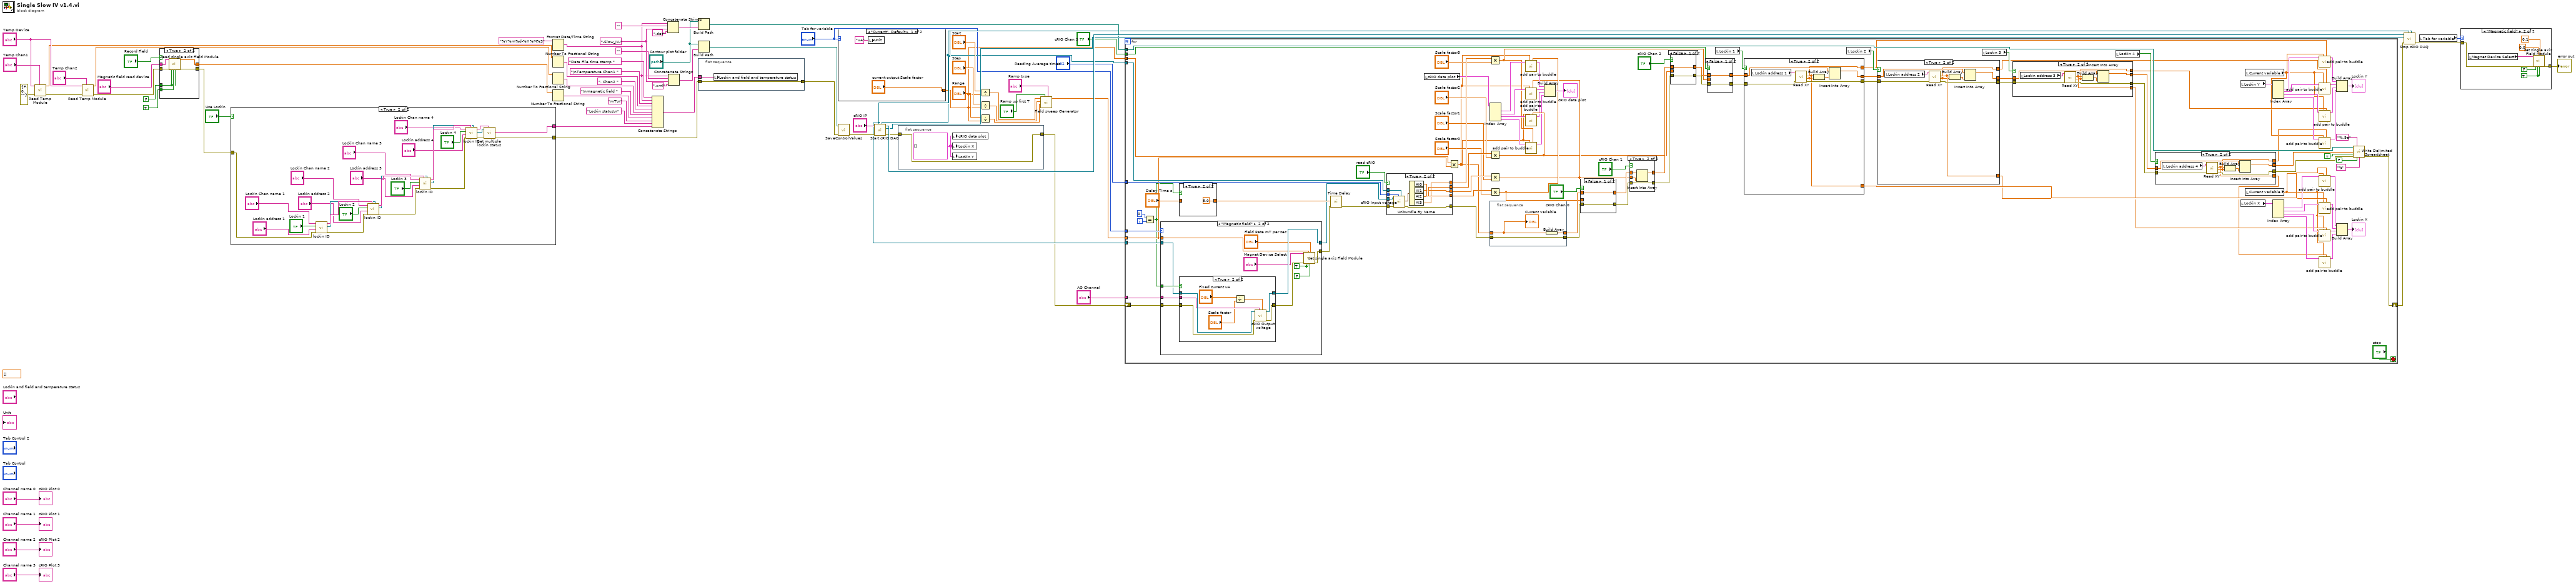
[diagram p0: block diagram]
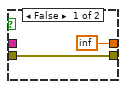
[diagram p2: hidden frame]
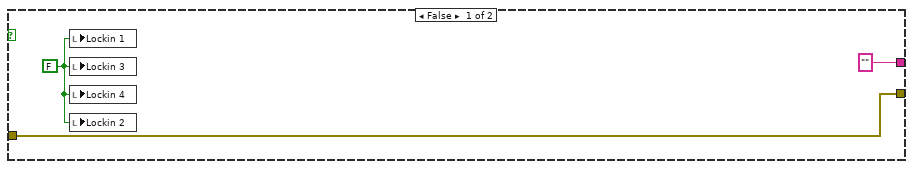
[diagram p3: hidden frame]
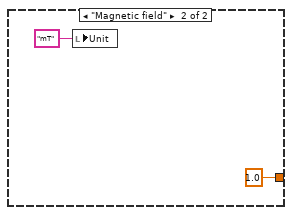
[diagram p5: hidden frame]
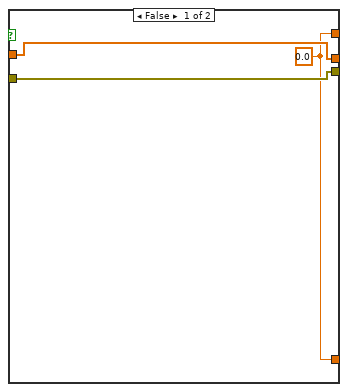
[diagram p6: hidden frame]
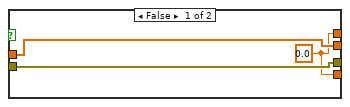
[diagram p7: hidden frame]
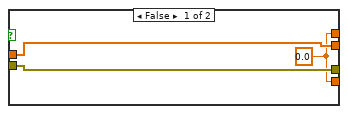
[diagram p8: hidden frame]
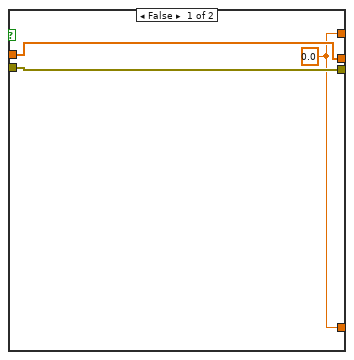
[diagram p9: hidden frame]
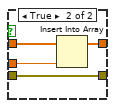
[diagram p10: hidden frame]
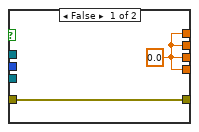
[diagram p11: hidden frame]
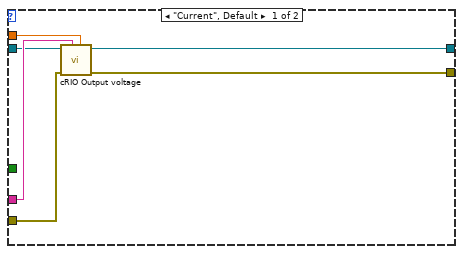
[diagram p12: hidden frame]
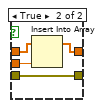
[diagram p15: hidden frame]
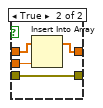
[diagram p16: hidden frame]
diagram:
  (unwired) dbl[] []
  w64 = "-Slow_IV-"
  n1 = call "Read Temp Module.vi"("Temp Chan"="Temp Chan1", "error in (no error)"=errorcluster {"status"=FALSE, "code"=0, "source"=""} ("error in"), "Device"="Temp Device") -> ("error out"=w31:errorcluster, "Temperature K"=w26:dbl)  [unwired: 7 in]
  n2 = call "Read Temp Module.vi"("Temp Chan"="Temp Chan2", "error in (no error)"=w31, "Device"="Temp Device") -> ("error out"=w24:errorcluster, "Temperature K"=w25:dbl)  [unwired: 7 in]
  n3 = case shown="True" "Record Field" {
    tunnel: w24 -> [w72 w78]
    tunnel: "Magnetic field read device" -> [_ w77]
    tunnel: [inf w76] -> w22
    tunnel: TRUE ("Exec") -> [_ w75]
    tunnel: FALSE ("Init") -> [_ w74]
    tunnel: [w72 w73] -> w7
    frame False {
    }
    frame True {
      n4 = call "read single axis Field Module.vi"("Magnet Device Select"=w77, "error in (no error)"=w78, "Init"=w74, "Exec"=w75, "final"=w74) -> ("FIeld mT"=w76:dbl, "error out"=w73:errorcluster)  [unwired: 13 in]
    }
  }
  n5 = case shown="True" "Use Lockin" {
    tunnel: ["" ("Status output") w108] -> w8
    tunnel: [w81 w107] -> w6
    tunnel: w7 -> [w81 w105]
    frame False {
      w79 = FALSE ("Lockin 1")
      n6 = local write "Lockin 1"(w79) -> ()
      n7 = local write "Lockin 3"(w79) -> ()
      n8 = local write "Lockin 4"(w79) -> ()
      n9 = local write "Lockin 2"(w79) -> ()
    }
    frame True {
      n10 = call "lockin ID.vi"("error in (no error)"=w105, "Lockin address"="Lockin address 1", "Lockin on"="Lockin 1", "Lockin Chan name"="Lockin Chan name 1") -> ("error out"=w98:errorcluster, "Addresses out"=w101:refnum<visa-resource-name>[], "names out"=w102:string[])  [unwired: 5 in]
      n11 = call "lockin ID.vi"("Addresses IN"=w101, "names in"=w102, "error in (no error)"=w98, "Lockin address"="Lockin address 2", "Lockin on"="Lockin 2", "Lockin Chan name"="Lockin Chan name 2") -> ("error out"=w94:errorcluster, "Addresses out"=w95:refnum<visa-resource-name>[], "names out"=w96:string[])  [unwired: 3 in]
      n12 = call "lockin ID.vi"("Addresses IN"=w95, "names in"=w96, "error in (no error)"=w94, "Lockin address"="Lockin address 3", "Lockin on"="Lockin 3", "Lockin Chan name"="Lockin Chan name 3") -> ("error out"=w90:errorcluster, "Addresses out"=w88:refnum<visa-resource-name>[], "names out"=w89:string[])  [unwired: 3 in]
      n13 = call "lockin ID.vi"("Addresses IN"=w88, "names in"=w89, "error in (no error)"=w90, "Lockin address"="Lockin address 4", "Lockin on"="Lockin 4", "Lockin Chan name"="Lockin Chan name 4") -> ("error out"=w82:errorcluster, "Addresses out"=w83:refnum<visa-resource-name>[], "names out"=w84:string[])  [unwired: 3 in]
      n14 = call "get multiple lockin status.vi"("Device channel names"=w84, "error in (no error)"=w82, "SRS830 addresses"=w83) -> ("error out"=w107:errorcluster, "Status output"=w108:string)  [unwired: 6 in, 1 out]
    }
  }
  n15 = Format Date/Time String(time format string (%c)="%Y%m%d-%H%M%S") -> (date/time string=w18:string)  [unwired: 2 in]
  n16 = Number To Fractional String(number=w26) -> (F-format string=w15:string)  [unwired: 3 in]
  n17 = Number To Fractional String(number=w25) -> (F-format string=w14:string)  [unwired: 3 in]
  n18 = Number To Fractional String(number=w22) -> (F-format string=w12:string)  [unwired: 3 in]
  n19 = Concatenate Strings("Data File time stamp " ("string"), w18, "\nTemperature Chan1 " ("string"), w15, ", Chan2 " ("string"), w14, "\nmagnetic field " ("string"), w12, "mT\n" ("string"), "Lockin status\n" ("string"), w8) -> (w4:string)
  n20 = Concatenate Strings(w18, "" ("string"), w64, ".dat" ("string")) -> (w66:string)
  n21 = Concatenate Strings(w18, "" ("string"), w64, ".xml" ("string")) -> (w69:string)
  n22 = Build Path(base path="Contour plot folder", name or relative path=w66) -> (appended path=w49:path)
  n23 = Build Path(base path="Contour plot folder", name or relative path=w69) -> (appended path=w67:path)
  n24 = flat-sequence {
    tunnel: w6 -> [w110]
    tunnel: [w110] -> w5
    tunnel: w4 -> [w109]
    frame #0 {
      n25 = local write "Lockin and field and temperature status"(w109) -> ()
    }
  }
  n26 = case shown="\"Current\", Default" "Tab for variable" {
    tunnel: ["current output Scale factor" 1.0 ("current output Scale factor")] -> w35
    frame "Current", Default {
      n27 = local write "Unit"("uA" ("Unit")) -> ()
    }
    frame "Magnetic field" {
      n28 = local write "Unit"("mT" ("Unit")) -> ()
    }
  }
  n29 = call "SaveControlValues.vi"("XML File Path"=w67, "error in (no error)"=w5) -> ("error out"=w62:errorcluster)  [unwired: 8 in]
  n30 = call "Start cRIO DAQ.vi"("error in (no error)"=w62, "cRIO IP"="cRIO IP") -> ("error out"=w2:errorcluster, "vi reference"=w60:refnum<vi>, "application reference"=w61:refnum<vi>, "DAQ_AI_Reader endpoint"=w47:refnum<k21>, "DAQ_CMD_Writer endpoint"=w48:refnum<k21>)  [unwired: 5 in]
  n31 = flat-sequence {
    tunnel: w2 -> [w116]
    tunnel: [w116] -> w1
    frame #0 {
      w115 = cluster{dbl[], dbl[]}[] [] ("appended array")
      n32 = local write "cRIO data plot"(w115) -> ()
      n33 = local write "Lockin X"(w115) -> ()
      n34 = local write "Lockin Y"(w115) -> ()
    }
  }
  n35 = Divide(x="Start", y=w35) -> (x/y=w37:dbl)
  n36 = Divide(x="Step", y=w35) -> (x/y=w53:dbl)
  n37 = Divide(x="Range", y=w35) -> (x/y=w52:dbl)
  n38 = call "Field sweep Generator.vi"("Ramp type"="Ramp type", "Ramp up first T"="Ramp up first T", "Field Radius"=w52, "Field step"=w53, "Field Origin"=w37) -> ("output array"=w50:dbl[])  [unwired: 6 in]
  n39 = for {
    tunnel: w48 -> [w189]
    tunnel: "AO Channel" -> [w190]
    tunnel: w50 -> [w191] mode=indexing
    tunnel: w47 -> [w220]
    tunnel: w49 -> [w219]
    tunnel: "cRIO Chan 3" -> [w205]
    tunnel: "Reading Average times" -> [w198]
    tunnel: "Tab for variable" -> [w192]
    tunnel: w35 -> [w185]
    shift-right: [w199] -> w43
    shift-left: w1 -> [w179]
    i -> [w196]
    stop <- "stop" stop-if-true
    n40 = Equal?(x=0, y=w196) -> (x = y?=w186:bool)
    n41 = case shown="\"Magnetic field\"" w192 {
      tunnel: w191 -> [w288 w292]
      tunnel: w190 -> [w287 w296]
      tunnel: w179 -> [w286 w299]
      tunnel: w189 -> [w285 w298]
      tunnel: [w284 w294] -> w188
      tunnel: [w283 w297] -> w187
      tunnel: w186 -> [_ w300]
      frame "Current", Default {
        n42 = call "cRIO Output voltage.vi"("Voltage"=w288, "AO Channel"=w287, "error in (no error)"=w286, "DAQ_CMD_Writer endpoint"=w285) -> ("error out"=w284:errorcluster, "DAQ_CMD_Writer endpoint out"=w283:refnum<k21>)  [unwired: 6 in]
      }
      frame "Magnetic field" {
        w290 = TRUE ("Init")
        n43 = case shown="True" w300 {
          tunnel: w299 -> [w301 w310]
          tunnel: [w301 w309] -> w295
          tunnel: w298 -> [w302 w308]
          tunnel: [w302 w307] -> w297
          tunnel: w296 -> [_ w306]
          frame False {
          }
          frame True {
            n44 = Divide(x="Fixed current uA", y="Scale factor") -> (x/y=w304:dbl)
            n45 = call "cRIO Output voltage.vi"("Voltage"=w304, "AO Channel"=w306, "error in (no error)"=w310, "DAQ_CMD_Writer endpoint"=w308) -> ("error out"=w309:errorcluster, "DAQ_CMD_Writer endpoint out"=w307:refnum<k21>)  [unwired: 6 in]
          }
        }
        n46 = call "set single axis Field Module.vi"("Magnet Device Select"="Magnet Device Select", "error in (no error)"=w295, "Init"=w290, "Field Target mT"=w292, "Exec"=w290, "Field Rate mT per sec"="Field Rate mT per sec", "final"=FALSE ("Exec")) -> ("error out"=w294:errorcluster)  [unwired: 12 in]
      }
    }
    n47 = case shown="True" w186 {
      tunnel: "Delay Time s" -> [w311 _]
      tunnel: [w311 5.0 ("Delay Time s")] -> w193
      frame False {
      }
      frame True {
      }
    }
    n48 = call "Time Delay"("error in (no error)"=w188, "Delay Time (s)"=w193) -> ("error out"=w215:errorcluster)  [unwired: 9 in]
    n49 = case shown="True" "read cRIO" {
      tunnel: w220 -> [_ w282]
      tunnel: w215 -> [w271 w281]
      tunnel: [w272 w279] -> w214
      tunnel: [w272 w278] -> w213
      tunnel: [w272 w277] -> w212
      tunnel: [w272 w276] -> w211
      tunnel: [w271 w275] -> w202
      tunnel: w198 -> [_ w274]
      tunnel: w187 -> [_ w273]
      frame False {
        w272 = 0.0 ("AI2")
      }
      frame True {
        n50 = call "cRIO Input voltage.vi"("DAQ_AI_Reader endpoint"=w282, "Average"=w274, "error in (no error)"=w281, "DAQ_CMD_Writer endpoint"=w273) -> ("error out"=w275:errorcluster, "output cluster"=w280:T1)  [unwired: 5 in, 1 out]
        n51 = Unbundle By Name(w280) -> ("AI0"=w279:dbl, "AI1"=w278:dbl, "AI2"=w277:dbl, "AI3"=w276:dbl)
      }
    }
    n52 = local read "cRIO data plot"() -> (w162:cluster{"Y":dbl[], "Y":dbl[]}[])
    n53 = Multiply(x=w185, y=w191) -> (x*y=w122:dbl)
    n54 = Multiply(x=w211, y="Scale factor3") -> (x*y=w150:dbl)
    n55 = Multiply(x=w212, y="Scale factor2") -> (x*y=w153:dbl)
    n56 = Multiply(x=w213, y="Scale factor1") -> (x*y=w155:dbl)
    n57 = Multiply(x=w214, y="Scale factor0") -> (x*y=w158:dbl)
    n58 = Index Array(array=w162) -> (element #1=w161:cluster{"Y":dbl[], "Y":dbl[]}, element #2=w157:cluster{"Y":dbl[], "Y":dbl[]}, element #3=w154:cluster{"Y":dbl[], "Y":dbl[]}, element #4=w151:cluster{"Y":dbl[], "Y":dbl[]})  [unwired: 4 in]
    n59 = flat-sequence {
      tunnel: w202 -> [w315]
      tunnel: [w315] -> w182
      tunnel: [w314] -> w183
      tunnel: w122 -> [w313]
      frame #0 {
        n60 = Build Array(w313) -> (w314:dbl[])
        "Current variable" <- w313
      }
    }
    n61 = call "add pair to buddle.vi"("y"=w158, "x"=w122, "Input"=w161) -> ("output"=w159:cluster{dbl[], dbl[]})  [unwired: 8 in]
    n62 = call "add pair to buddle.vi"("y"=w155, "x"=w122, "Input"=w157) -> ("output"=w156:cluster{dbl[], dbl[]})  [unwired: 8 in]
    n63 = call "add pair to buddle.vi"("y"=w153, "x"=w122, "Input"=w154) -> ("output"=w152:cluster{dbl[], dbl[]})  [unwired: 8 in]
    n64 = call "add pair to buddle.vi"("y"=w150, "x"=w122, "Input"=w151) -> ("output"=w149:cluster{dbl[], dbl[]})  [unwired: 8 in]
    n65 = Build Array(w159, w156, w152, w149) -> (→"cRIO data plot":cluster{dbl[], dbl[]}[])
    n66 = case shown="False" "cRIO Chan 0" {
      tunnel: w182 -> [w265 w270]
      tunnel: [w265 w270] -> w181
      tunnel: w183 -> [w266 w269]
      tunnel: w158 -> [_ w268]
      tunnel: [w266 w267] -> w180
      frame False {
      }
      frame True {
        n67 = Insert Into Array(array=w269, new element=w268) -> (w267:dbl[])  [unwired: 1 in]
      }
    }
    n68 = case shown="True" "cRIO Chan 1" {
      tunnel: w181 -> [w328 w333]
      tunnel: [w328 w333] -> w204
      tunnel: w180 -> [w329 w332]
      tunnel: w155 -> [_ w331]
      tunnel: [w329 w330] -> w201
      frame False {
      }
      frame True {
        n69 = Insert Into Array(array=w332, new element=w331) -> (w330:dbl[])  [unwired: 1 in]
      }
    }
    n70 = case shown="False" "cRIO Chan 2" {
      tunnel: w204 -> [w322 w327]
      tunnel: [w322 w327] -> w203
      tunnel: w201 -> [w323 w326]
      tunnel: w153 -> [_ w325]
      tunnel: [w323 w324] -> w200
      frame False {
      }
      frame True {
        n71 = Insert Into Array(array=w326, new element=w325) -> (w324:dbl[])  [unwired: 1 in]
      }
    }
    n72 = case shown="False" w205 {
      tunnel: w203 -> [w316 w318]
      tunnel: w200 -> [w317 w321]
      tunnel: w150 -> [_ w320]
      tunnel: [w317 w319] -> w165
      tunnel: [w316 w318] -> w172
      frame False {
      }
      frame True {
        n73 = Insert Into Array(array=w321, new element=w320) -> (w319:dbl[])  [unwired: 1 in]
      }
    }
    n74 = local read "Lockin 1"() -> (w169:bool)
    n75 = case shown="True" w169 {
      tunnel: w172 -> [w222 w228]
      tunnel: [w222 w227] -> w177
      tunnel: w165 -> [w223 w230]
      tunnel: [w223 w231] -> w178
      tunnel: [w221 w225] -> w145
      tunnel: [w221 w224] -> w130
      frame False {
        w221 = 0.0 ("Y mV")
      }
      frame True {
        n76 = local read "Lockin address 1"() -> (w229:string)
        n77 = call "Read XY.vi"("error in (no error)"=w228, "VISA resource name"=w229) -> ("error out"=w227:errorcluster, "Y mV"=w224:dbl, "X mV"=w225:dbl)  [unwired: 6 in, 1 out]
        n78 = Build Array(w225, w224) -> (w226:dbl[])
        n79 = Insert Into Array(array=w230, new element=w226) -> (w231:dbl[])  [unwired: 1 in]
      }
    }
    n80 = local read "Lockin 2"() -> (w168:bool)
    n81 = case shown="True" w168 {
      tunnel: w177 -> [w255 w262]
      tunnel: [w255 w261] -> w173
      tunnel: w178 -> [w256 w259]
      tunnel: [w256 w260] -> w175
      tunnel: [w254 w258] -> w141
      tunnel: [w254 w257] -> w128
      frame False {
        w254 = 0.0 ("Y mV")
      }
      frame True {
        n82 = local read "Lockin address 2"() -> (w263:string)
        n83 = call "Read XY.vi"("error in (no error)"=w262, "VISA resource name"=w263) -> ("error out"=w261:errorcluster, "Y mV"=w257:dbl, "X mV"=w258:dbl)  [unwired: 6 in, 1 out]
        n84 = Build Array(w258, w257) -> (w264:dbl[])
        n85 = Insert Into Array(array=w259, new element=w264) -> (w260:dbl[])  [unwired: 1 in]
      }
    }
    n86 = local read "Lockin 3"() -> (w167:bool)
    n87 = case shown="True" w167 {
      tunnel: w173 -> [w244 w251]
      tunnel: [w244 w248] -> w174
      tunnel: w175 -> [w245 w250]
      tunnel: [w245 w249] -> w176
      tunnel: [w243 w247] -> w140
      tunnel: [w243 w246] -> w126
      frame False {
        w243 = 0.0 ("X mV")
      }
      frame True {
        n88 = local read "Lockin address 3"() -> (w252:string)
        n89 = call "Read XY.vi"("error in (no error)"=w251, "VISA resource name"=w252) -> ("error out"=w248:errorcluster, "Y mV"=w246:dbl, "X mV"=w247:dbl)  [unwired: 6 in, 1 out]
        n90 = Build Array(w247, w246) -> (w253:dbl[])
        n91 = Insert Into Array(array=w250, new element=w253) -> (w249:dbl[])  [unwired: 1 in]
      }
    }
    n92 = local read "Lockin 4"() -> (w166:bool)
    n93 = case shown="True" w166 {
      tunnel: w174 -> [w233 w240]
      tunnel: w176 -> [w234 w237]
      tunnel: [w234 w238] -> w163
      tunnel: [w233 w239] -> w171
      tunnel: [w232 w236] -> w139
      tunnel: [w232 w235] -> w124
      frame False {
        w232 = 0.0 ("X mV")
      }
      frame True {
        n94 = local read "Lockin address 4"() -> (w241:string)
        n95 = call "Read XY.vi"("error in (no error)"=w240, "VISA resource name"=w241) -> ("error out"=w239:errorcluster, "Y mV"=w235:dbl, "X mV"=w236:dbl)  [unwired: 6 in, 1 out]
        n96 = Build Array(w236, w235) -> (w242:dbl[])
        n97 = Insert Into Array(array=w237, new element=w242) -> (w238:dbl[])  [unwired: 1 in]
      }
    }
    n98 = local read "Lockin Y"() -> (w135:cluster{"Y":dbl[], "Y":dbl[]}[])
    n99 = local read "Lockin X"() -> (w148:cluster{"Y":dbl[], "Y":dbl[]}[])
    n100 = local read "Current variable"() -> (w120:dbl)
    n101 = local read "Current variable"() -> (w121:dbl)
    n102 = Index Array(array=w135) -> (element #1=w134:cluster{"Y":dbl[], "Y":dbl[]}, element #2=w133:cluster{"Y":dbl[], "Y":dbl[]}, element #3=w132:cluster{"Y":dbl[], "Y":dbl[]}, element #4=w131:cluster{"Y":dbl[], "Y":dbl[]})  [unwired: 4 in]
    n103 = Index Array(array=w148) -> (element #1=w147:cluster{"Y":dbl[], "Y":dbl[]}, element #2=w144:cluster{"Y":dbl[], "Y":dbl[]}, element #3=w143:cluster{"Y":dbl[], "Y":dbl[]}, element #4=w142:cluster{"Y":dbl[], "Y":dbl[]})  [unwired: 4 in]
    n104 = call "add pair to buddle.vi"("y"=w130, "x"=w120, "Input"=w134) -> ("output"=w129:cluster{dbl[], dbl[]})  [unwired: 8 in]
    n105 = call "add pair to buddle.vi"("y"=w128, "x"=w120, "Input"=w133) -> ("output"=w127:cluster{dbl[], dbl[]})  [unwired: 8 in]
    n106 = call "add pair to buddle.vi"("y"=w126, "x"=w120, "Input"=w132) -> ("output"=w125:cluster{dbl[], dbl[]})  [unwired: 8 in]
    n107 = call "add pair to buddle.vi"("y"=w124, "x"=w120, "Input"=w131) -> ("output"=w123:cluster{dbl[], dbl[]})  [unwired: 8 in]
    n108 = call "add pair to buddle.vi"("y"=w145, "x"=w121, "Input"=w147) -> ("output"=w146:cluster{dbl[], dbl[]})  [unwired: 8 in]
    n109 = call "add pair to buddle.vi"("y"=w141, "x"=w121, "Input"=w144) -> ("output"=w138:cluster{dbl[], dbl[]})  [unwired: 8 in]
    n110 = call "add pair to buddle.vi"("y"=w140, "x"=w121, "Input"=w143) -> ("output"=w137:cluster{dbl[], dbl[]})  [unwired: 8 in]
    n111 = call "add pair to buddle.vi"("y"=w139, "x"=w121, "Input"=w142) -> ("output"=w136:cluster{dbl[], dbl[]})  [unwired: 8 in]
    n112 = Build Array(w129, w127, w125, w123) -> (→"Lockin Y":cluster{dbl[], dbl[]}[])
    n113 = Build Array(w146, w138, w137, w136) -> (→"Lockin X":cluster{dbl[], dbl[]}[])
    n114 = call-poly <vilib>:"Write Delimited Spreadsheet.vi"("file path (dialog if empty)"=w219, "format (%.3f)"="%.9e", "1D data"=w163, "append to file? (new file:F)"=TRUE, "error in (no error)"=w171, "transpose? (no:F)"=FALSE, "delimiter (\\t)"="\t" ("delimiter (\\t)")) -> ("error out"=w199:errorcluster)  [unwired: 7 in, 1 out]
  }
  n115 = call "Stop cRIO DAQ.vi"("DAQ_AI_Reader endpoint"=w47, "DAQ_CMD_Writer endpoint"=w48, "error in (no error)"=w43, "VI reference"=w60, "application reference"=w61) -> ("error out"=w33:errorcluster)  [unwired: 6 in]
  n116 = local read "Tab for variable"() -> (w34:enum32{"Current", "Magnetic field"})
  n117 = case shown="\"Magnetic field\"" w34 {
    tunnel: w33 -> [w334 w338]
    tunnel: [w334 w337] -> w32
    frame "Current", Default {
    }
    frame "Magnetic field" {
      w335 = TRUE ("Exec")
      n118 = local read "Magnet Device Select"() -> (w341:string)
      n119 = call "set single axis Field Module.vi"("Magnet Device Select"=w341, "error in (no error)"=w338, "Init"=FALSE, "Field Target mT"=0.0, "Exec"=w335, "Field Rate mT per sec"=0.1, "final"=w335) -> ("error out"=w337:errorcluster)  [unwired: 12 in]
    }
  }
  "error out" <- w32
  "cRIO Plot 0" <- "Channel name 0"
  "cRIO Plot 1" <- "Channel name 1"
  "cRIO Plot 2" <- "Channel name 2"
  "cRIO Plot 3" <- "Channel name 3"
